vi "icListen 2 Enabled.vi"() -> ()   [LabVIEW 2020, in "PAM Library.lvlib"]
uses:
  PAM Library.lvlib
panel:
  in  "icListen 2 Enabled":bool
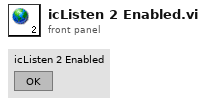
[diagram p1: front panel]
diagram:
